vi "AutoInit.vi"   [LabVIEW 2019]
doc: "Set all robot instructions to their proper intial state."
uses:
  dscommands.vi
  autoninfo.vi
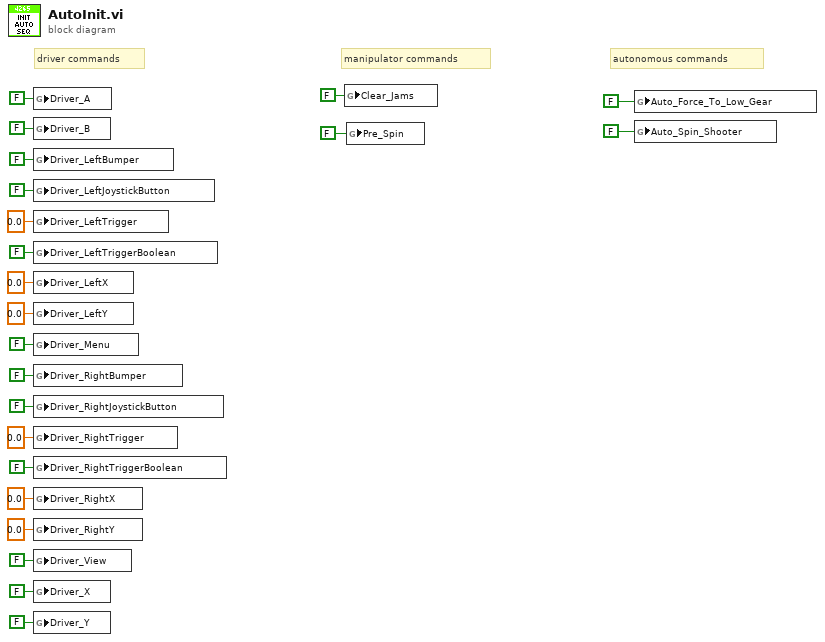
[diagram p0: block diagram]
diagram:
  # "manipulator commands"
  # "driver commands"
  # "autonomous commands"
  n1 = global write "dscommands.vi" "Driver_A"(FALSE ("Driver_A")) -> ()
  n2 = global write "dscommands.vi" "Driver_B"(FALSE ("Driver_B")) -> ()
  n3 = global write "dscommands.vi" "Driver_LeftBumper"(FALSE ("Driver_LeftBumper")) -> ()
  n4 = global write "dscommands.vi" "Driver_LeftJoystickButton"(FALSE ("Driver_LeftJoystickButton")) -> ()
  n5 = global write "dscommands.vi" "Driver_LeftTrigger"(0.0 ("Driver_LeftTrigger")) -> ()
  n6 = global write "dscommands.vi" "Driver_LeftTriggerBoolean"(FALSE ("Driver_LeftTriggerBoolean")) -> ()
  n7 = global write "dscommands.vi" "Driver_LeftX"(0.0 ("Driver_LeftX")) -> ()
  n8 = global write "dscommands.vi" "Driver_LeftY"(0.0 ("Driver_LeftY")) -> ()
  n9 = global write "dscommands.vi" "Driver_Menu"(FALSE ("Driver_Menu")) -> ()
  n10 = global write "dscommands.vi" "Driver_RightBumper"(FALSE ("Driver_RightBumper")) -> ()
  n11 = global write "dscommands.vi" "Driver_RightJoystickButton"(FALSE ("Driver_RightJoystickButton")) -> ()
  n12 = global write "dscommands.vi" "Driver_RightTrigger"(0.0 ("Driver_RightTrigger")) -> ()
  n13 = global write "dscommands.vi" "Driver_RightTriggerBoolean"(FALSE ("Driver_RightTriggerBoolean")) -> ()
  n14 = global write "dscommands.vi" "Driver_RightX"(0.0 ("Driver_RightX")) -> ()
  n15 = global write "dscommands.vi" "Driver_RightY"(0.0 ("Driver_RightY")) -> ()
  n16 = global write "dscommands.vi" "Driver_View"(FALSE ("Driver_View")) -> ()
  n17 = global write "dscommands.vi" "Driver_X"(FALSE ("Driver_X")) -> ()
  n18 = global write "dscommands.vi" "Driver_Y"(FALSE ("Driver_Y")) -> ()
  n19 = global write "dscommands.vi" "Clear_Jams"(FALSE ("Clear_Jams")) -> ()
  n20 = global write "dscommands.vi" "Pre_Spin"(FALSE ("Clear_Jams")) -> ()
  n21 = global write "autoninfo.vi" "Auto_Force_To_Low_Gear"(FALSE ("Auto_Force_To_Low_Gear")) -> ()
  n22 = global write "autoninfo.vi" "Auto_Spin_Shooter"(FALSE ("Auto_Force_To_Low_Gear")) -> ()
